vi "保存文件.vi"(8 "Title数据整合输入":string[](array[string]), 11 "路径原始":path) -> (3 "路径输出":path)   [LabVIEW 2011]
uses:
  <vilib>/Utility/file.llb/Read From Spreadsheet File (string).vi
  <vilib>/Utility/file.llb/Write To Spreadsheet File (string).vi
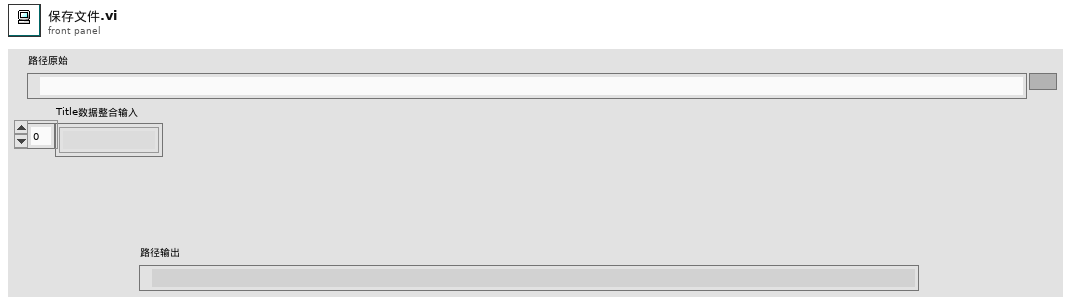
[diagram p1: front panel]
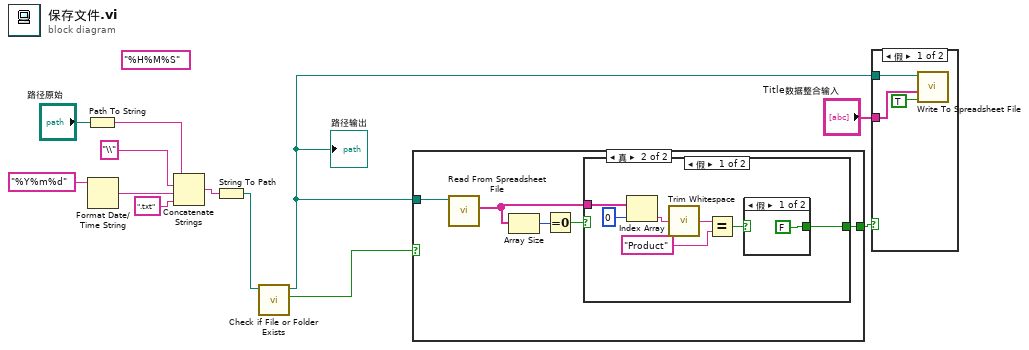
[diagram p0: block diagram]
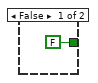
[diagram p2: hidden frame]
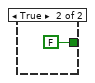
[diagram p4: hidden frame]
diagram:
  (unwired) "%H%M%S" ("时间格式字符串(%c)")
  n1 = Path To String(path="路径原始") -> (string=w3:string)
  n2 = Format Date/Time String(time format string (%c)="%Y%m%d" ("时间格式字符串(%c)")) -> (date/time string=w11:string)  [unwired: 2 in]
  n3 = Concatenate Strings(w3, "\\" ("字符串"), w11, ".txt" ("字符串")) -> (w2:string)
  n4 = String To Path(string=w2) -> (path=w1:path)
  n5 = call <vilib>:"Check if File or Folder Exists.vi"("path"=w1) -> ("file or folder exists?"=w6:bool, "dup path"=w5:path)  [unwired: 8 in, 1 out]
  "路径输出" <- w5
  n6 = case shown="真" w6 {
    tunnel: w5 -> [_ w18]
    tunnel: [FALSE w17] -> w8
    frame False {
    }
    frame True {
      n7 = call-poly <vilib>:"Read From Spreadsheet File.vi"("file path (dialog if empty)"=w18) -> ("first row"=w14:string[])  [unwired: 6 in, 4 out]
      n8 = Array Size(array=w14) -> (size(s)=w16:i32)
      n9 = Equal To 0?(x=w16) -> (x = 0?=w15:bool)
      n10 = case shown="假" w15 {
        tunnel: [w21 FALSE] -> w17
        tunnel: w14 -> [w23 _]
        frame False {
          n11 = Index Array(array=w23, index=0 ("索引 (行)")) -> (element=w24:string)
          n12 = call <vilib>:"Trim Whitespace.vi"("string"=w24) -> ("trimmed string"=w20:string)  [unwired: 1 in]
          n13 = Equal?(x=w20, y="Product" ("trimmed string")) -> (x = y?=w22:bool)
          n14 = case shown="假" w22 {
            selector: w22 -> [_ w27]
            tunnel: [FALSE w27] -> w21
            frame False {
            }
            frame True {
            }
          }
        }
        frame True {
        }
      }
    }
  }
  n15 = case shown="假" w8 {
    tunnel: w5 -> [w30 _]
    tunnel: "Title数据整合输入" -> [w29 _]
    frame False {
      n16 = call-poly <vilib>:"Write To Spreadsheet File.vi"("append to file? (new file:F)"=TRUE, "1D data"=w29, "file path (dialog if empty)"=w30) -> ()  [unwired: 5 in, 1 out]
    }
    frame True {
    }
  }
